vi "NotifierDestory.vi"   [LabVIEW 2014]
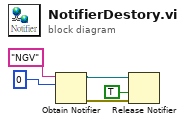
[diagram p0: block diagram]
diagram:
  n1 = Obtain Notifier(name (unnamed)="NGV", notification data type=0 ("Numeric")) -> (notifier out=w2:refnum<notifier>, error out=w3:errorcluster)  [unwired: 2 in, 1 out]
  n2 = Release Notifier(notifier=w2, force destroy? (F)=TRUE, error in (no error)=w3) -> ()  [unwired: 3 out]
